vi "createAll.vi"(8 "error in (no error)":errorcluster, 11 "SAL_Events in":refnum<class "SAL_Events.lvclass">) -> (0 "error out":errorcluster, 3 "SAL_Events out":refnum<class "SAL_Events.lvclass">)   [LabVIEW 2016, in "SAL_Events.lvclass"]
uses:
  SAL_Events.lvclass
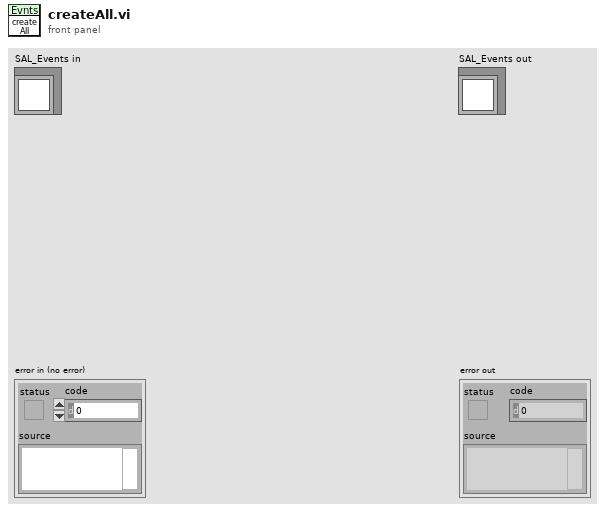
[diagram p1: front panel]
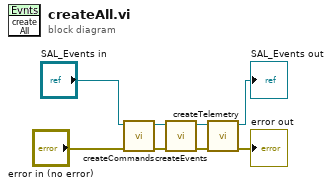
[diagram p0: block diagram]
diagram:
  n1 = call "createCommands.vi"("error in (no error)"="error in (no error)", "SAL_Events in"="SAL_Events in") -> ("error out"=w6:errorcluster, "SAL_Events out"=w8:refnum<class "SAL_Events.lvclass">)  [unwired: 8 in]
  n2 = call "createEvents.vi"("error in (no error)"=w6, "SAL_Events in"=w8) -> ("error out"=w5:errorcluster, "SAL_Events out"=w7:refnum<class "SAL_Events.lvclass">)  [unwired: 8 in]
  n3 = call "createTelemetry.vi"("error in (no error)"=w5, "SAL_Events in"=w7) -> ("error out"=→"error out":errorcluster, "SAL_Events out"=→"SAL_Events out":refnum<class "SAL_Events.lvclass">)  [unwired: 8 in]
